vi "AMLUTwaveselect.vi"(1 "Wave Shape":u8(ring) items=["Sine", "Ramp", "Triangle"], 3 "LUTsize":u8=32) -> (0 "Array":u8[](array[numeric])=[0, 4, 8, 12, 16, 20, 24, 28, 32, 35, 39, 43, 47, 51, 55, 59, 63, 59, 55, 51, 47, 43, 39, 35, 32, 28, 24, 20, 16, 12, 8, 4])   [LabVIEW 2017]
panel:
  # "Create Wave shapes for AM\nfrom 0-63 in amplitude and\nlength of LUTsize"
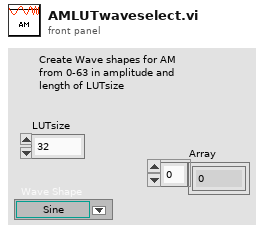
[diagram p1: front panel]
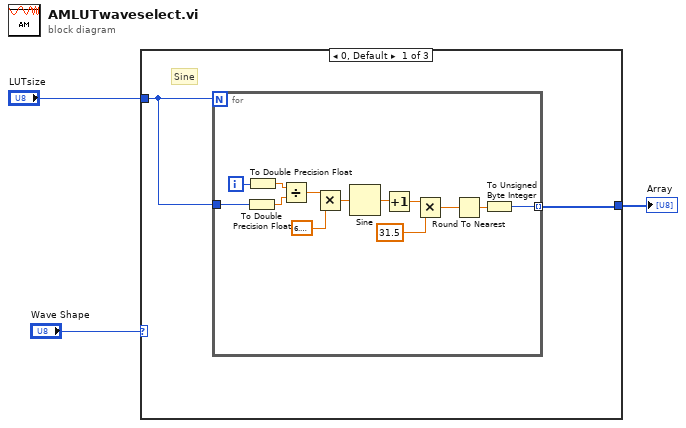
[diagram p0: block diagram]
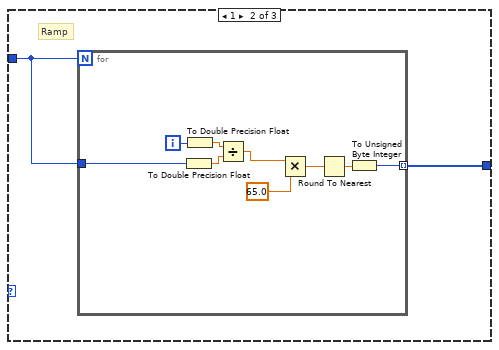
[diagram p2: hidden frame]
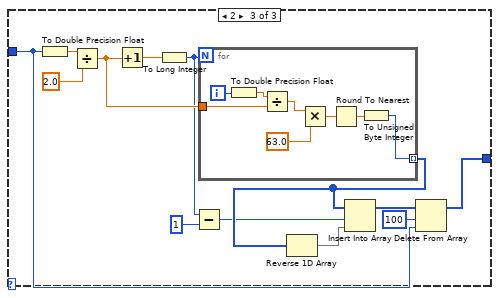
[diagram p3: hidden frame]
diagram:
  n1 = case shown="0, Default" "Wave Shape" {
    tunnel: [w4 w20 w32] -> w1
    tunnel: "LUTsize" -> [w5 w19 w31]
    frame 0, Default {
      # "Sine"
      n2 = for {
        N: w5 -> [_]
        tunnel: [w10] -> w4 mode=indexing
        tunnel: w5 -> [w6]
        i -> [w14]
        n3 = To Double Precision Float(number=w6) -> (double precision float=w12:dbl)
        n4 = To Double Precision Float(number=w14) -> (double precision float=w13:dbl)
        n5 = Divide(x=w13, y=w12) -> (x/y=w18:dbl)
        n6 = Multiply(x=w18, y=6.283185307179586) -> (x*y=w16:dbl)
        n7 = Sine(x=w16) -> (sin(x)=w15:dbl)
        n8 = Increment(x=w15) -> (x+1=w9:dbl)
        n9 = Multiply(x=w9, y=31.5) -> (x*y=w7:dbl)
        n10 = Round To Nearest(number=w7) -> (nearest integer value=w11:dbl)
        n11 = To Unsigned Byte Integer(number=w11) -> (unsigned 8bit integer=w10:u8)
      }
    }
    frame 1 {
      # "Ramp"
      n12 = for {
        N: w19 -> [_]
        tunnel: [w25] -> w20 mode=indexing
        tunnel: w19 -> [w22]
        i -> [w29]
        n13 = To Double Precision Float(number=w22) -> (double precision float=w27:dbl)
        n14 = To Double Precision Float(number=w29) -> (double precision float=w28:dbl)
        n15 = Divide(x=w28, y=w27) -> (x/y=w21:dbl)
        n16 = Multiply(x=w21, y=65.0) -> (x*y=w23:dbl)
        n17 = Round To Nearest(number=w23) -> (nearest integer value=w26:dbl)
        n18 = To Unsigned Byte Integer(number=w26) -> (unsigned 8bit integer=w25:u8)
      }
    }
    frame 2 {
      n19 = To Double Precision Float(number=w31) -> (double precision float=w42:dbl)
      n20 = Divide(x=w42, y=2.0) -> (x/y=w37:dbl)
      n21 = Increment(x=w37) -> (x+1=w38:dbl)
      n22 = To Long Integer(number=w38) -> (32bit integer=w36:i32)
      n23 = Subtract(x=w36, y=1) -> (x-y=w35:i32)
      n24 = for {
        N: w36 -> [_]
        tunnel: [w44] -> w40 mode=indexing
        tunnel: w37 -> [w43]
        i -> [w45]
        n25 = To Double Precision Float(number=w45) -> (double precision float=w46:dbl)
        n26 = Divide(x=w46, y=w43) -> (x/y=w50:dbl)
        n27 = Multiply(x=w50, y=63.0) -> (x*y=w49:dbl)
        n28 = Round To Nearest(number=w49) -> (nearest integer value=w47:dbl)
        n29 = To Unsigned Byte Integer(number=w47) -> (unsigned 8bit integer=w44:u8)
      }
      n30 = Reverse 1D Array(array=w40) -> (reversed array=w39:u8[])
      n31 = Insert Into Array(array=w40, index=w35, new element=w39) -> (w33:u8[])
      n32 = Delete From Array(array=w33, length=100, index=w31) -> (array with subset deleted=w32:u8[])  [unwired: 1 out]
    }
  }
  "Array" <- w1
